vi "toml_read_int.vi"(5 "action":T3, 6 "options in":T1, 7 "section":string[](array[string]), 8 "error in (no error)":errorcluster, 9 "default":i64, 10 "key":string[](array[string]), 11 "path in":path) -> (0 "error out":errorcluster, 1 "value":i64, 2 "exists?":bool, 3 "path out":path, 4 "options out":T1)   [LabVIEW 2017]
uses:
  toml_key_action.ctl
  toml_int_format.ctl
  toml_int_options.ctl
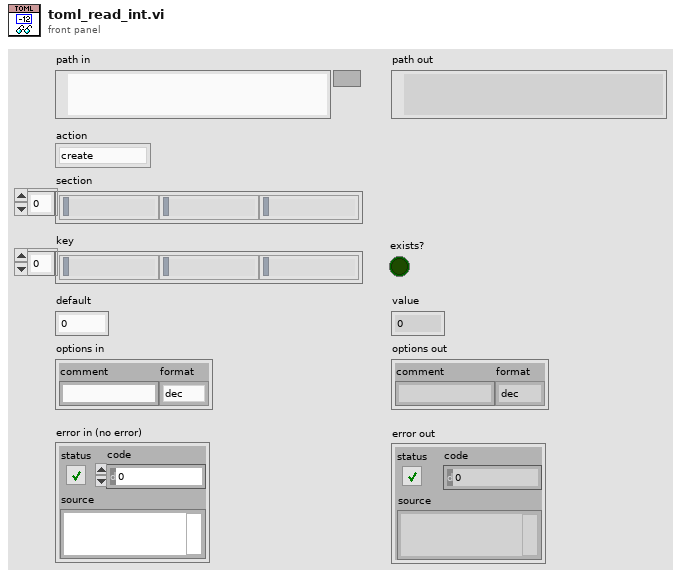
[diagram p1: front panel]
types:
  T1 = typedef "toml_int_options.ctl" = cluster{"comment":string, "format":T2}
  T2 = typedef "toml_int_format.ctl" = enum8{"dec", "hex", "oct", "bin"}
  T3 = typedef "toml_key_action.ctl" = enum8{"create", "read", "write", "delete"}
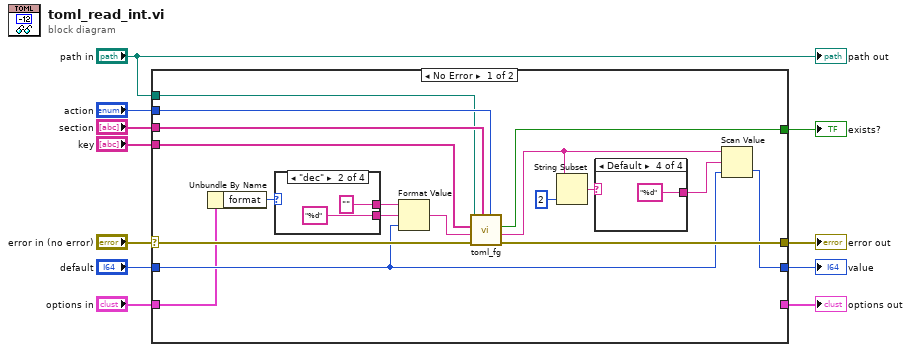
[diagram p0: block diagram]
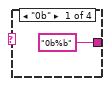
[diagram p2: hidden frame]
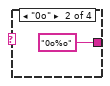
[diagram p3: hidden frame]
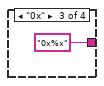
[diagram p4: hidden frame]
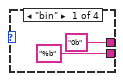
[diagram p5: hidden frame]
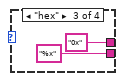
[diagram p6: hidden frame]
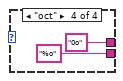
[diagram p7: hidden frame]
diagram:
  n1 = case shown="No Error" "error in (no error)" {
    selector: "error in (no error)" -> [w27 w44]
    tunnel: "section" -> [w29 _]
    tunnel: "key" -> [w28 _]
    tunnel: "default" -> [w18 w43]
    tunnel: [w21 w44] -> w10
    tunnel: [w26 _] -> w9
    tunnel: "action" -> [w25 _]
    tunnel: "path in" -> [w24 _]
    tunnel: [w19 w43] -> w3
    tunnel: "options in" -> [w13 w42]
    tunnel: [_ w42] -> w1
    frame No Error {
      n2 = Unbundle By Name(w13) -> ("format"=w12:T2)
      n3 = case shown="\"dec\"" w12 {
        tunnel: ["%b" ("format string") "%d" ("format string") "%x" ("format string") "%o" ("format string")] -> w17
        tunnel: ["0b" ("string (\"\")") "" ("string (\"\")") "0x" ("string (\"\")") "0o" ("string (\"\")")] -> w16
        frame "bin" {
        }
        frame "dec" {
        }
        frame "hex" {
        }
        frame "oct" {
        }
      }
      n4 = Format Value(string ("")=w16, format string=w17, value (0)=w18) -> (output string=w20:string)
      n5 = call "toml_fg.vi"("action"=w25, "section"=w29, "error in (no error)"=w27, "value in"=w20, "key"=w28, "path in"=w24) -> ("error out"=w21:errorcluster, "value out"=w22:string, "exists?"=w26:bool)  [unwired: 1 in, 2 out]
      n6 = String Subset(string=w22, length (rest)=2 ("length (rest)")) -> (substring=w14:string)  [unwired: 1 in]
      n7 = case shown="Default" w14 {
        tunnel: ["0b%b" ("format string") "0o%o" ("format string") "0x%x" ("format string") "%d" ("format string")] -> w15
        frame "0b" {
        }
        frame "0o" {
        }
        frame "0x" {
        }
        frame Default {
        }
      }
      n8 = Scan Value(string=w22, format string=w15, default (0 dbl)=w18) -> (value=w19:i64)  [unwired: 1 out]
    }
    frame Error {
    }
  }
  "error out" <- w10
  "value" <- w3
  "exists?" <- w9
  "options out" <- w1
  "path out" <- "path in"
